vi "setNext.vi"(8 "error in (no error)":errorcluster, 10 "next":refnum<data-value>, 11 "LLNode in":refnum<class "LLNode.lvclass">) -> (0 "error out":errorcluster, 3 "LLNode out":refnum<class "LLNode.lvclass">)   [LabVIEW 2014, in "LinkedList.lvlib" / "LLNode.lvclass"]
doc: "Sets the Node next in the linked list."
uses:
  <userlib>/AdvancedDataStructures/ClassBased/LLNode/LLNode.lvclass
  <userlib>/AdvancedDataStructures/ClassBased/LLNode/LLNode.lvclass/LLNode.ctl
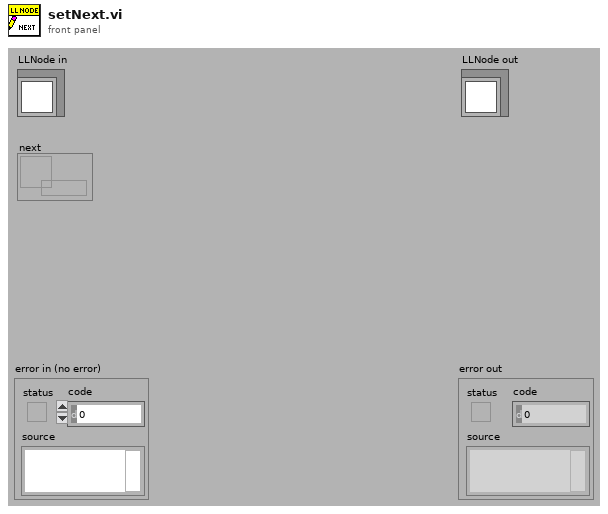
[diagram p1: front panel]
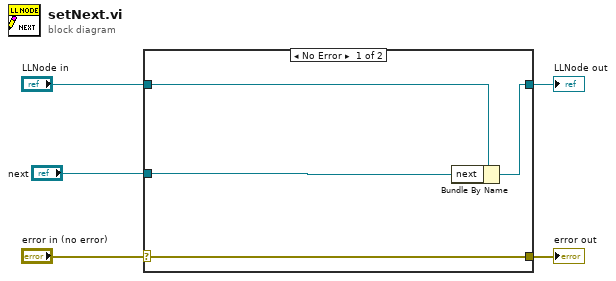
[diagram p0: block diagram]
diagram:
  n1 = case shown="No Error" "error in (no error)" {
    selector: "error in (no error)" -> [w9 w10]
    tunnel: [w9 w10] -> w4
    tunnel: [w7 w11] -> w2
    tunnel: "LLNode in" -> [w8 w11]
    tunnel: "next" -> [w6 _]
    frame No Error {
      n2 = Bundle By Name(cluster=w8, "next"=w6) -> (w7:refnum<class "LLNode.lvclass">)
    }
    frame Error {
    }
  }
  "error out" <- w4
  "LLNode out" <- w2
